vi "PH_Beamline.PC Clear beamline.vi"(0 "i ref in":refnum<vi>, 5 "error IO":errorcluster) -> (14 "i ref out":refnum<vi>, 19 "error out":errorcluster)   [LabVIEW 2014, in "PH_Beamline.lvlib"]
doc: "This is the Proc case \"Clear Beamline\"."
uses:
  PH_Beamline.lvlib
  PH_Beamline.Switch Instances.ctl
  PH_Basics/PH_StatusHandler/PH_StatusHandler.Status.ctl
  PH_Beamline.Black Box Instances.ctl
  PH_Beamline.6P Switch Instances.ctl
  PH_Classes/PH_Switch/PH_Switch.lvlib
  PH_Basics/PH_StatusHandler/PH_StatusHandler.lvlib
  PH_Motion/PH_Sixpack_Switch/PH_Sixpack_Switch.lvlib
  PH_BL-Master/PH_BL-Master.lvlib
  PH_Classes/PH_BlackBox/PH_BlackBox.lvlib
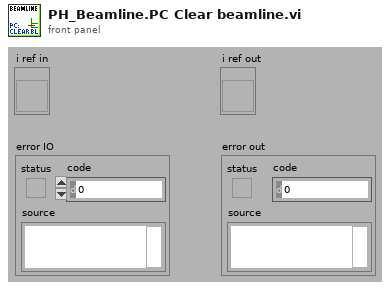
[diagram p1: front panel]
types:
  T1 = typedef "PH_Beamline.lvlib/PH_Beamline.Black Box Instances.ctl" = string
  T2 = typedef "PH_Beamline.lvlib/PH_Beamline.6P Switch Instances.ctl" = string
  T3 = typedef "PH_Beamline.lvlib/PH_Beamline.Switch Instances.ctl" = string
  T4 = typedef "PH_StatusHandler.lvlib/PH_StatusHandler.Status.ctl" = i16
  T5 = typedef "PH_Beamline.lvlib/PH_Beamline.i attribute.ctl" = cluster{"GUI Refs":cluster{"PA ok":refnum<vi>, "MA ok":refnum<vi>, "fs FE ok":refnum<vi>, "ns FE ok":refnum<vi>, "PA ED ok":refnum<vi>, "MAS ok":refnum<vi>, "Booster ok":refnum<vi>, "Mirrortower ok":refnum<vi>, "In.-Box ok":refnum<vi>, "Compressor ok":refnum<vi>, "Experiment LB ok":refnum<vi>, "Experiment LL ok":refnum<vi>, "PHELIX_Beckhoff_Watchdog":refnum<vi>, "Shutters closed":refnum<vi>, "uOPA ok":refnum<vi>, "Vacuum no shotcond Comp LB":refnum<vi>}, "Refs BL MA":refnum<vi>[], "Refs BL MA-IB":refnum<vi>[], "Refs BL fs":refnum<vi>[], "Refs BL PA ED":refnum<vi>[], "Refs BL MAS":refnum<vi>[], "Refs BL Boo":refnum<vi>[], "Refs BL ns":refnum<vi>[], "Refs BL Mirrortower":refnum<vi>[], "Refs BL Compressor":refnum<vi>[], "Refs BL Exp LB":refnum<vi>[], "Radiation Safety":cluster{"Exp Laserbay":cluster{"Ref Op Mode":refnum<vi>, "Ref Laserbay evacuated":refnum<vi>, "Tagname LB evacuated":string, "Shot Mode":T6, "Laserbay evacuated?":i32, "Tagname HV room locked":string, "HV room locked?":i32, "Ref HV room locked":refnum<vi>, "Tagname bridged?":string, "Ref Bridge":refnum<vi>, "I<1E18W/cm²":bool}, "Exp Laserlab":cluster{"Ref Op Mode":refnum<vi>, "Ref Laserlab evacuated":refnum<vi>, "Tagname LL evacuated":string, "Shot Mode":T6, "Laserlab evacuated?":i32, "Tagname bridged?":string, "Ref Bridge":refnum<vi>, "I<1E18W/cm²":bool}}, "Refs BL LL":refnum<vi>[], "PP Igni Heating GUI Refs":refnum<vi>[], "PP Igni Heating Tagnames ":string[], "Refs BL PA":cluster{"undelayed Line before Shutter":refnum<vi>[], "undelayed Line after Shutter":refnum<vi>[], "before Bypass":refnum<vi>[], "delayed Line before Shutter":refnum<vi>[], "delayed Line after Shutter":refnum<vi>[], "before Shutter Input":refnum<vi>[], "after Shutter Input":refnum<vi>[], "Bypass":refnum<vi>[], "before Shutter Exit":refnum<vi>[], "after Shutter Exit":refnum<vi>[], "to MA":refnum<vi>[], "to Lab":refnum<vi>[]}, "BL":cluster{"YLF_BL_Status":i32, "fs_BL_Status":i32, "fs_YLF_BL_Status":i32, "ns_BL_Status":i32, "PA_Input_BL_Status":i32, "PA_UnDelay_BL_Status":i32, "PA_Delay_BL_Status":i32, "PA_BL_Status":i32, "PA_Bypass_BL_Status":i32, "PA_Exit_BL_Status":i32, "PA_LL_BL_Status":i32, "LL_BL_Status":i32, "PA_MA_BL_Status":i32, "MA_Exit_BL_Status":i32, "MA_Z6_BL_Status":i32, "Z6_BL_Status":i32, "MA_LB_BL_Status":i32, "LB_TB2_BL_Status":i32, "PA_before_Bypass_BL_Status":i32, "LB_TB3_BL_Status":i32}, "State Subsystems":cluster{"PA":bool, "MA":bool, "ns FE":bool, "fs FE":bool, "PA ED":bool, "In.-Box":bool, "MAS":bool, "Booster":bool, "Mirrortower":bool, "Compressor":bool, "Experiment LB":bool, "Experiment LL":bool, "uOPA":bool}, "Status Subscriber Information":T7, "Refs BL uOPA":refnum<vi>[], "PA_Input_2_Beam_6PWpGUI not linked?":bool, "PA_Input_Delay_6PGUI not linked?":bool, "Settings":T10}
  T6 = typedef "PH_Beamline.lvlib/PH_Beamline.Operation Mode.ctl" = i32
  T7 = typedef "PH_Beamline.lvlib/PH_Beamline.Status Subscriber Information.ctl" = cluster{"fs Swich YLF":T8, "fs Exit Shutter":T8, "ns Exit Shutter":T8, "PA Input Shutter":T8, "PA PC WP":T8, "PA PC WP 2":T8, "PA Bypass In":T8, "PA Bypass Out":T8, "PA CH 1":T8, "PA delayed":T8, "PA non delayed":T8, "PA Exit Shutter":T8, "PA Switch Lab":T8, "PA Bridge CH Input MA":T8, "MA Diffusor IB":T8, "MA IB Ready":T8, "MA CH 1":T8, "MA CH 2":T8, "MA CH 3":T8, "MA CH 4":T8, "MA Shutter Align Cam":T8, "MA Position MM5":T8, "Calorimeter Switch":T8, "BL Z6 CH 9":T8, "BL Z6 Beamdump":T8, "BL Z6 Shutter":T8, "COS Sensitivity Switch":T8, "Exp LB Shutter":T8, "Exp LB TB 2":T8, "Exp LB TB 3":T8, "PA LL Input CH":T8, "PA LL Output CH":T8, "LL Comp Input Shutter":T8, "LL Comp Output Shutter":T8, "LL Comp FF Shutter":T8, "Exp LL Shutter":T8, "MA IM In IB":T8, "MA IM Out IB":T8, "MA DB In IB":T8, "MA DB Out IB":T8, "Exp LB Shutter Interlock":T8, "Exp LL Shutter Interlock":T8, "MM1 Force Sensor":T8}
  T8 = typedef "PH_BL-Master.lvlib/PH_BL-Master.Status Subscriber Information.ctl" = cluster{"Index of element":i32, "Attributeset":T9}
  T9 = typedef "PH_BL-Master.lvlib/PH_BL-Master.Attribute Set.ctl" = enum16{"Boolean Status Service Subscriber", "Picture Status Service Subscriber"}
  T10 = typedef "PH_Beamline_Chief.lvlib/PH_Beamline_Chief.Settings.ctl" = cluster{"PA Doublepass Mode":bool, "Compressor Vaccuum LB not relevant":bool, "Windowshutter TB2 not relevant":bool, "Windowshutter TB3 not relevant":bool}
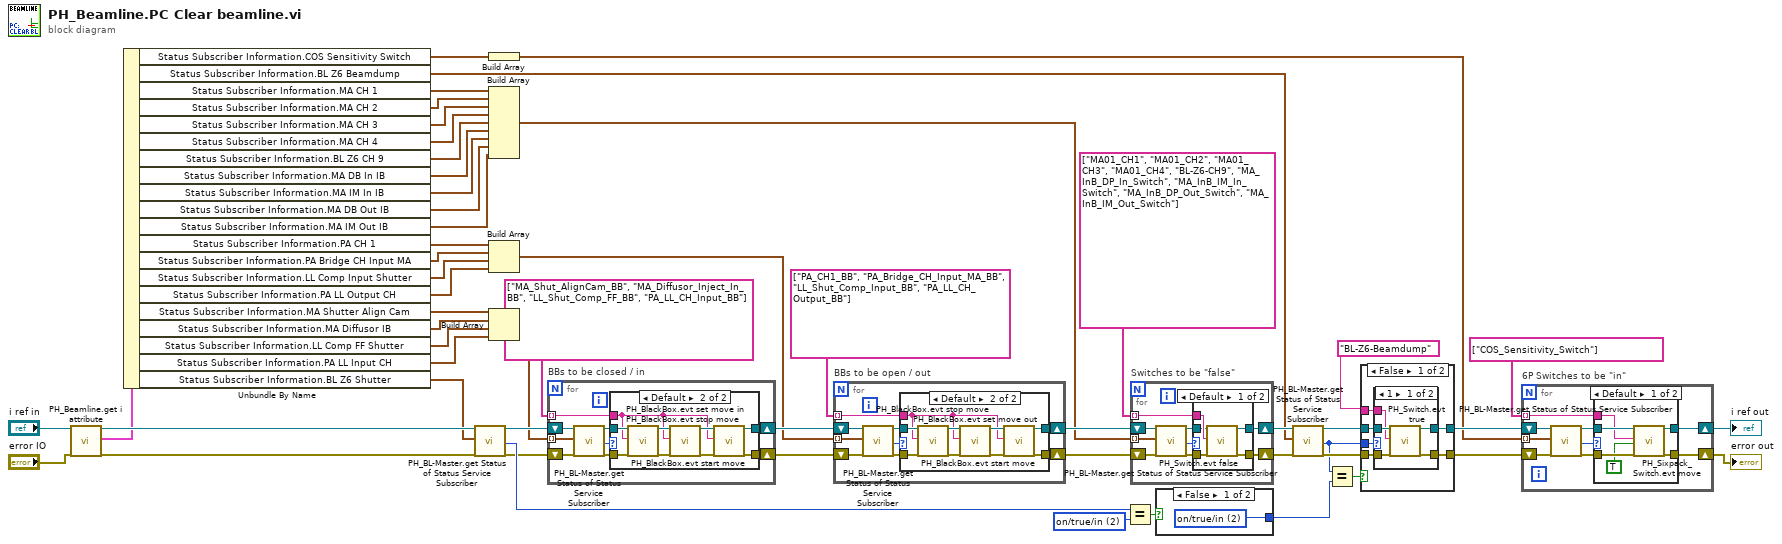
[diagram p0: block diagram]
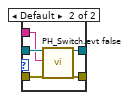
[diagram p3: hidden frame]
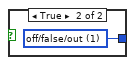
[diagram p5: hidden frame]
diagram:
  w49 = T4 2 items=["no info", "off/false/out", "on/true/in", "Failure", "Alarm", "Status 1", "Status 2", "Status 3"] ("y")
  n1 = call "PH_Beamline.get i attribute.vi"("i ref in"="i ref in", "error in (no error)"="error IO") -> ("i ref out"=w26:refnum<vi>, "i attribute"=w25:T5, "error out"=w28:errorcluster)  [unwired: 15 in]
  n2 = Unbundle By Name(w25) -> ("Status Subscriber Information.COS Sensitivity Switch"=w2:T8, "Status Subscriber Information.BL Z6 Beamdump"=w3:T8, "Status Subscriber Information.MA CH 1"=w13:T8, "Status Subscriber Information.MA CH 2"=w12:T8, "Status Subscriber Information.MA CH 3"=w11:T8, "Status Subscriber Information.MA CH 4"=w10:T8, "Status Subscriber Information.BL Z6 CH 9"=w9:T8, "Status Subscriber Information.MA DB In IB"=w8:T8, "Status Subscriber Information.MA IM In IB"=w7:T8, "Status Subscriber Information.MA DB Out IB"=w6:T8, "Status Subscriber Information.MA IM Out IB"=w5:T8, "Status Subscriber Information.PA CH 1"=w18:T8, "Status Subscriber Information.PA Bridge CH Input MA"=w17:T8, "Status Subscriber Information.LL Comp Input Shutter"=w16:T8, "Status Subscriber Information.PA LL Output CH"=w15:T8, "Status Subscriber Information.MA Shutter Align Cam"=w23:T8, "Status Subscriber Information.MA Diffusor IB"=w22:T8, "Status Subscriber Information.LL Comp FF Shutter"=w21:T8, "Status Subscriber Information.PA LL Input CH"=w20:T8, "Status Subscriber Information.BL Z6 Shutter"=w24:T8)
  n3 = call "PH_BL-Master.get Status of Status Service Subscriber.vi"("i ref in"=w26, "Wanted Status Subscriber Information"=w24, "error in (no error)"=w28) -> ("i ref out"=w41:refnum<vi>, "Status"=w52:T4, "error out"=w40:errorcluster)  [unwired: 11 in, 3 out]
  n4 = Build Array(w2) -> (w1:T8[])
  n5 = Build Array(w13, w12, w11, w10, w9, w8, w7, w6, w5) -> (w4:T8[])
  n6 = Build Array(w18, w17, w16, w15) -> (w14:T8[])
  n7 = Build Array(w23, w22, w21, w20) -> (w19:T8[])
  n8 = for "BBs to be closed / in" {
    tunnel: T1[] ["MA_Shut_AlignCam_BB", "MA_Diffusor_Inject_In_BB", "LL_Shut_Comp_FF_BB", "PA_LL_CH_Input_BB"] -> [w56] mode=indexing
    shift-right: [w59] -> w37
    shift-left: w41 -> [w60]
    shift-right: [w57] -> w38
    shift-left: w40 -> [w58]
    tunnel: w19 -> [w55] mode=indexing
    n9 = call "PH_BL-Master.get Status of Status Service Subscriber.vi"("i ref in"=w60, "Wanted Status Subscriber Information"=w55, "error in (no error)"=w58) -> ("i ref out"=w62:refnum<vi>, "Status"=w61:T4, "error out"=w63:errorcluster)  [unwired: 11 in, 3 out]
    n10 = case shown="Default" w61 {
      tunnel: w62 -> [w65 w70]
      tunnel: [w65 w69] -> w59
      tunnel: w63 -> [w64 w68]
      tunnel: [w64 w67] -> w57
      tunnel: w56 -> [_ w66]
      frame 2 {
      }
      frame Default {
        n11 = call "PH_BlackBox.evt stop move.vi"("i ref in"=w70, "Instance"=w66, "error in (no error)"=w68) -> ("i ref out"=w74:refnum<vi>, "error out"=w73:errorcluster)  [unwired: 15 in]
        n12 = call "PH_BlackBox.evt set move in.vi"("i ref in"=w74, "Instance"=w66, "error in (no error)"=w73) -> ("i ref out"=w71:refnum<vi>, "error out"=w72:errorcluster)  [unwired: 15 in]
        n13 = call "PH_BlackBox.evt start move.vi"("i ref in"=w71, "Instance"=w66, "error in (no error)"=w72) -> ("i ref out"=w69:refnum<vi>, "error out"=w67:errorcluster)  [unwired: 15 in]
      }
    }
  }
  n14 = for "BBs to be open / out" {
    tunnel: T1[] ["PA_CH1_BB", "PA_Bridge_CH_Input_MA_BB", "LL_Shut_Comp_Input_BB", "PA_LL_CH_Output_BB"] -> [w76] mode=indexing
    shift-right: [w79] -> w36
    shift-left: w37 -> [w78]
    shift-right: [w80] -> w35
    shift-left: w38 -> [w77]
    tunnel: w14 -> [w75] mode=indexing
    n15 = call "PH_BL-Master.get Status of Status Service Subscriber.vi"("i ref in"=w78, "Wanted Status Subscriber Information"=w75, "error in (no error)"=w77) -> ("i ref out"=w82:refnum<vi>, "Status"=w81:T4, "error out"=w83:errorcluster)  [unwired: 11 in, 3 out]
    n16 = case shown="Default" w81 {
      tunnel: w82 -> [w85 w90]
      tunnel: [w85 w89] -> w79
      tunnel: w83 -> [w84 w88]
      tunnel: [w84 w87] -> w80
      tunnel: w76 -> [_ w86]
      frame 1 {
      }
      frame Default {
        n17 = call "PH_BlackBox.evt stop move.vi"("i ref in"=w90, "Instance"=w86, "error in (no error)"=w88) -> ("i ref out"=w94:refnum<vi>, "error out"=w93:errorcluster)  [unwired: 15 in]
        n18 = call "PH_BlackBox.evt set move out.vi"("i ref in"=w94, "Instance"=w86, "error in (no error)"=w93) -> ("i ref out"=w91:refnum<vi>, "error out"=w92:errorcluster)  [unwired: 15 in]
        n19 = call "PH_BlackBox.evt start move.vi"("i ref in"=w91, "Instance"=w86, "error in (no error)"=w92) -> ("i ref out"=w89:refnum<vi>, "error out"=w87:errorcluster)  [unwired: 15 in]
      }
    }
  }
  n20 = Equal?(x=w52, y=w49) -> (x = y?=w48:bool)
  n21 = for "Switches to be \"false\"" {
    shift-right: [w103] -> w50
    shift-left: w36 -> [w99]
    shift-right: [w102] -> w51
    shift-left: w35 -> [w101]
    tunnel: T3[] ["MA01_CH1", "MA01_CH2", "MA01_CH3", "MA01_CH4", "BL-Z6-CH9", "MA_InB_DP_In_Switch", "MA_InB_IM_In_Switch", "MA_InB_DP_Out_Switch", "MA_InB_IM_Out_Switch"] -> [w96] mode=indexing
    tunnel: w4 -> [w95] mode=indexing
    n22 = call "PH_BL-Master.get Status of Status Service Subscriber.vi"("i ref in"=w99, "Wanted Status Subscriber Information"=w95, "error in (no error)"=w101) -> ("i ref out"=w98:refnum<vi>, "Status"=w97:T4, "error out"=w100:errorcluster)  [unwired: 11 in, 3 out]
    n23 = case shown="Default" w97 {
      tunnel: w96 -> [w108 _]
      tunnel: [w107 w110] -> w103
      tunnel: w98 -> [w106 w110]
      tunnel: w100 -> [w105 w109]
      tunnel: [w104 w109] -> w102
      frame Default {
        n24 = call "PH_Switch.evt false.vi"("i ref in"=w106, "Instance"=w108, "error in (no error)"=w105) -> ("i ref out"=w107:refnum<vi>, "error out"=w104:errorcluster)  [unwired: 15 in]
      }
      frame 1 {
      }
    }
  }
  n25 = case shown="False" w48 {
    tunnel: [w111 w112] -> w47
    frame False {
      w111 = T4 2 items=["no info", "off/false/out", "on/true/in", "Failure", "Alarm", "Status 1", "Status 2", "Status 3"] ("x")
    }
    frame True {
      w112 = T4 1 items=["no info", "off/false/out", "on/true/in", "Failure", "Alarm", "Status 1", "Status 2", "Status 3"] ("x")
    }
  }
  n26 = call "PH_BL-Master.get Status of Status Service Subscriber.vi"("i ref in"=w50, "Wanted Status Subscriber Information"=w3, "error in (no error)"=w51) -> ("i ref out"=w45:refnum<vi>, "Status"=w43:T4, "error out"=w44:errorcluster)  [unwired: 11 in, 3 out]
  n27 = Equal?(x=w43, y=w47) -> (x = y?=w46:bool)
  n28 = case shown="False" w46 {
    tunnel: [w115 w130] -> w31
    tunnel: w45 -> [w117 w130]
    tunnel: w44 -> [w116 w129]
    tunnel: [w114 w129] -> w33
    tunnel: w43 -> [w118 _]
    tunnel: T3 "BL-Z6-Beamdump" ("Switch Instance") -> [w113 _]
    frame False {
      n29 = case shown="1" w118 {
        tunnel: w117 -> [w123 w127]
        tunnel: w116 -> [w122 w128]
        tunnel: [w121 w126] -> w115
        tunnel: [w120 w125] -> w114
        tunnel: w113 -> [w119 w124]
        frame 1 {
          n30 = call "PH_Switch.evt true.vi"("i ref in"=w123, "Instance"=w119, "error in (no error)"=w122) -> ("i ref out"=w121:refnum<vi>, "error out"=w120:errorcluster)  [unwired: 15 in]
        }
        frame Default {
          n31 = call "PH_Switch.evt false.vi"("i ref in"=w127, "Instance"=w124, "error in (no error)"=w128) -> ("i ref out"=w126:refnum<vi>, "error out"=w125:errorcluster)  [unwired: 15 in]
        }
      }
    }
    frame True {
    }
  }
  n32 = for "6P Switches to be \"in\"" {
    tunnel: T2[] ["COS_Sensitivity_Switch"] -> [w132] mode=indexing
    shift-right: [w134] -> w32
    shift-left: w31 -> [w138]
    shift-right: [w135] -> w34
    shift-left: w33 -> [w139]
    tunnel: w1 -> [w131] mode=indexing
    n33 = call "PH_BL-Master.get Status of Status Service Subscriber.vi"("i ref in"=w138, "Wanted Status Subscriber Information"=w131, "error in (no error)"=w139) -> ("i ref out"=w133:refnum<vi>, "Status"=w137:T4, "error out"=w136:errorcluster)  [unwired: 11 in, 3 out]
    n34 = case shown="Default" w137 {
      tunnel: w136 -> [w145 w146]
      tunnel: w133 -> [w144 w147]
      tunnel: [w143 w147] -> w134
      tunnel: [w142 w146] -> w135
      tunnel: w132 -> [w141 _]
      frame Default {
        n35 = call "PH_Sixpack_Switch.evt move.vi"("i ref in"=w144, "Instance"=w141, "Move"=TRUE, "error in (no error)"=w145) -> ("i ref out"=w143:refnum<vi>, "error out"=w142:errorcluster)  [unwired: 14 in]
      }
      frame 2 {
      }
    }
  }
  "error out" <- w34
  "i ref out" <- w32
